vi "grSim_ReplacementTester.vi"(0 "Generate new random points":bool, 1 "IA State":T3, 2 "Atacando contra?":bool, 3 "Test Attacker":bool, 4 "id":i32, 5 "Field defense":i32[](array[numeric]), 6 "Test Mode On":bool, 7 "Number of Points":i32, 9 "Região do campo\nTeste Passe":enum16{"3", "2", "1", "0", "-1", "-2", "-3"}(ring), 10 "Modulo Velocidade":dbl format="%#_13g", 11 "Test Passe":bool, 12 "reset":bool, 13 "Replace Robots":bool) -> (14 "grSim replacement":cluster{"robots":T1[], "ball":T2}, 15 "Replace active":bool, 16 "Number of goals":i16, 18 "kick num":i32, 19 "Completed Generation":bool)   [LabVIEW 2017]
uses:
  Core/AI Input.ctl
  Core/AI Robot.ctl
  Intel/Functions Enum.ctl
  Intel/AttackerStates.ctl
  Path Planning/RRT/PathDests.ctl
  Path Planning/RRT/PathDest.ctl
  Core/AI Ball.ctl
  Core/Field Size.ctl
  Core/AI Judge.ctl
  Intel/Command Enum.ctl
  Util/Events/Events.ctl
  grSim RobotReplacement.ctl
  grSim_BallReplacement.ctl
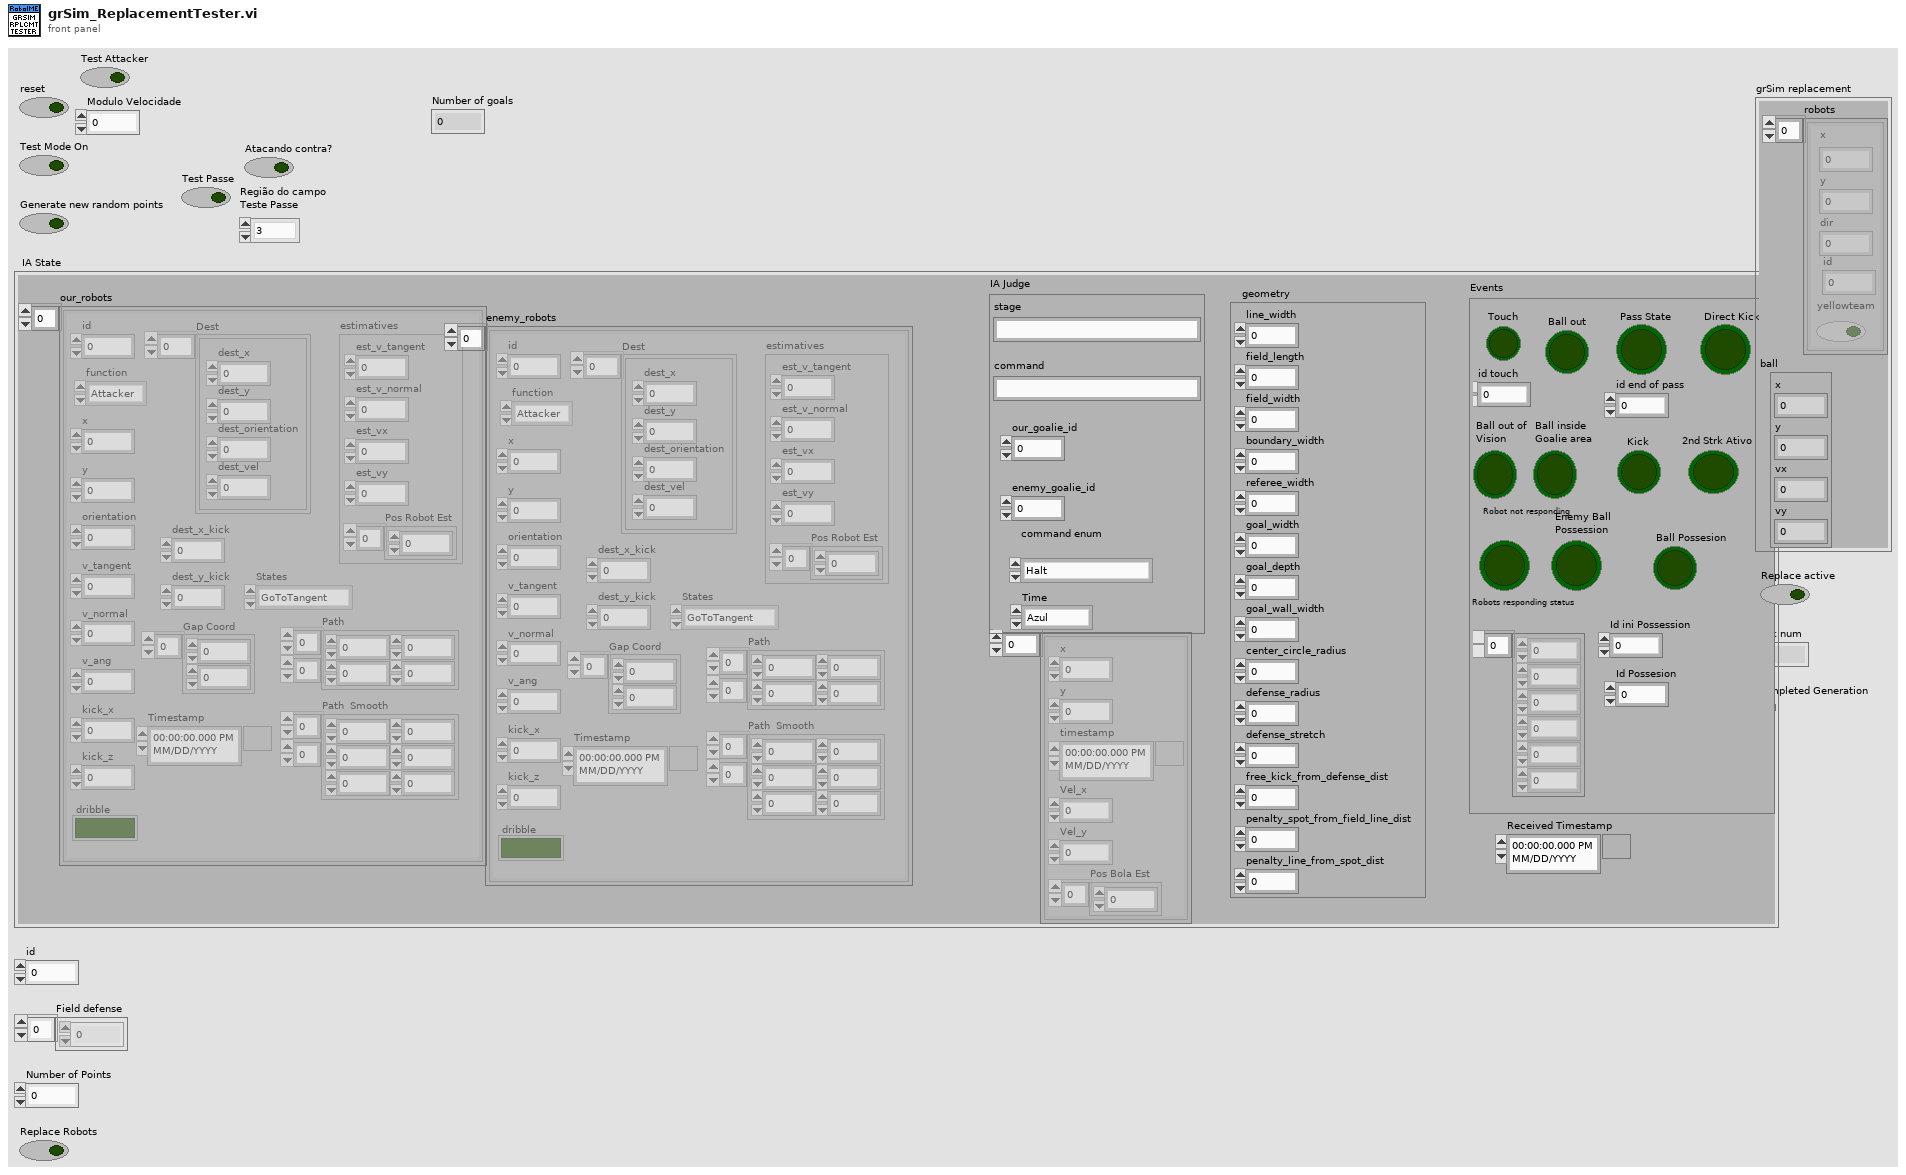
[diagram p1: front panel]
types:
  T1 = typedef "grSim RobotReplacement.ctl" = cluster{"x":dbl, "y":dbl, "dir":dbl, "yellowteam":bool, "id":u32}
  T2 = typedef "grSim_BallReplacement.ctl" = cluster{"x":dbl, "y":dbl, "vx":dbl, "vy":dbl}
  T3 = typedef "AI Input.ctl" = cluster{"our_robots":T4[], "enemy_robots":T4[], "balls":T9[], "geometry":T10, "IA Judge":T11, "Received Timestamp":timestamp, "Events":T13}
  T4 = typedef "AI Robot.ctl" = cluster{"id":u32, "function":T5, "x":dbl, "y":dbl, "orientation":dbl, "v_tangent":dbl, "v_normal":dbl, "v_ang":dbl, "kick_x":dbl, "kick_z":dbl, "dribble":bool, "Timestamp":timestamp, "estimatives":cluster{"est_v_tangent":dbl, "est_v_normal":dbl, "est_vx":dbl, "est_vy":dbl, "Pos Robot Est":dbl[]}, "dest_x_kick":dbl, "dest_y_kick":dbl, "Gap Coord":dbl[], "States":T6, "Path ":dbl[][], "Path  Smooth":dbl[][], "Dest":T7}
  T5 = typedef "Functions Enum.ctl" = enum16{"2nd Striker", "Attacker", "Goalie", "Defender", "Striker", "Goto 0", "Dummy", "Kicker", "ZigZag 0", "ZigZag 1", "ZigZag 2", "ZigZag 3", "ZigZag 4", "ZigZag 5", "ZigZag 6", "ZigZag 7", "ZigZag 8", ""}
  T6 = typedef "AttackerStates.ctl" = enum16{"Pass", "GoToTangent", "BallGetting", "GoToKick", ""}
  T7 = typedef "PathDests.ctl" = T8[]
  T8 = typedef "PathDest.ctl" = cluster{"dest_x":dbl, "dest_y":dbl, "dest_orientation":dbl, "dest_vel":dbl}
  T9 = typedef "AI Ball.ctl" = cluster{"x":dbl, "y":dbl, "timestamp":timestamp, "Vel_x":dbl, "Vel_y":dbl, "Pos Bola Est":dbl[]}
  T10 = typedef "Field Size.ctl" = cluster{"line_width":u32, "field_length":u32, "field_width":u32, "boundary_width":u32, "referee_width":u32, "goal_width":u32, "goal_depth":u32, "goal_wall_width":u32, "center_circle_radius":u32, "defense_radius":u32, "defense_stretch":u32, "free_kick_from_defense_dist":u32, "penalty_spot_from_field_line_dist":u32, "penalty_line_from_spot_dist":u32}
  T11 = typedef "AI Judge.ctl" = cluster{"stage":string, "command":string, "our_goalie_id":dbl, "enemy_goalie_id":dbl, "command enum":T12, "Time":enum16{"Azul", "Amarelo"}}
  T12 = typedef "Command Enum.ctl" = enum16{"Halt", "Stop", "Force Start", "PKA Normal Start", "Prepare Kickoff Ally", "PKE Normal Start", "Prepare Kickoff Enemy", "Prepare Penalty Ally", "PPA Normal Start", "Prepare Penalty Enemy", "PPE Normal Start", "Direct Free Enemy", "Direct Free Ally", "Indirect Free Enemy", "Indirect Free Ally", "Timeout Enemy", "Timeout Ally", "Goal Enemy", "Goal Ally", "Ball Placement Enemy", "Ball Placement Ally", "Normal Half Time", "Extra Time Break", "Extra Half Time", "None", "Post Game"}
  T13 = typedef "Events.ctl" = cluster{"Touch":bool, "Ball out":bool, "id touch":dbl, "Ball out of \nVision":bool, "Ball inside \nGoalie area":bool, "Robot not responding":bool, "Robots responding status":dbl[], "Enemy Ball \nPossession":bool, "Pass State":bool, "id end of pass":dbl, "Kick":bool, "Id ini Possession":dbl, "Ball Possesion":bool, "Id Possesion":dbl, "Direct Kick":bool, "2nd Strk Ativo":bool}
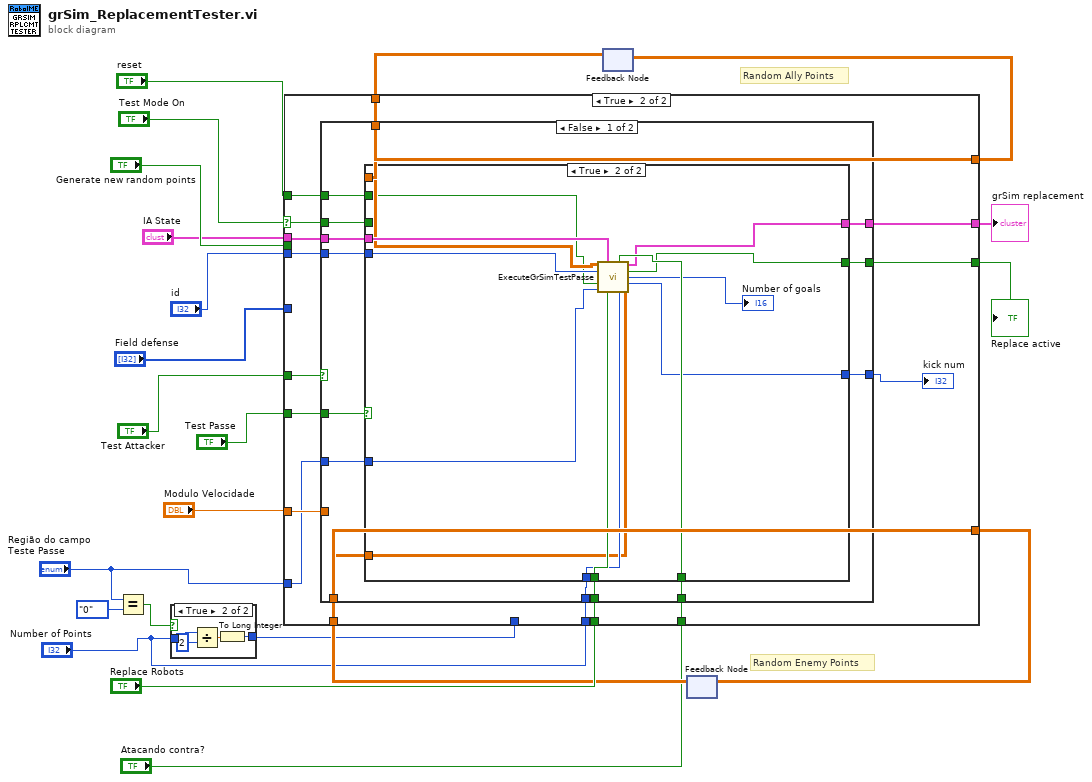
[diagram p0: block diagram]
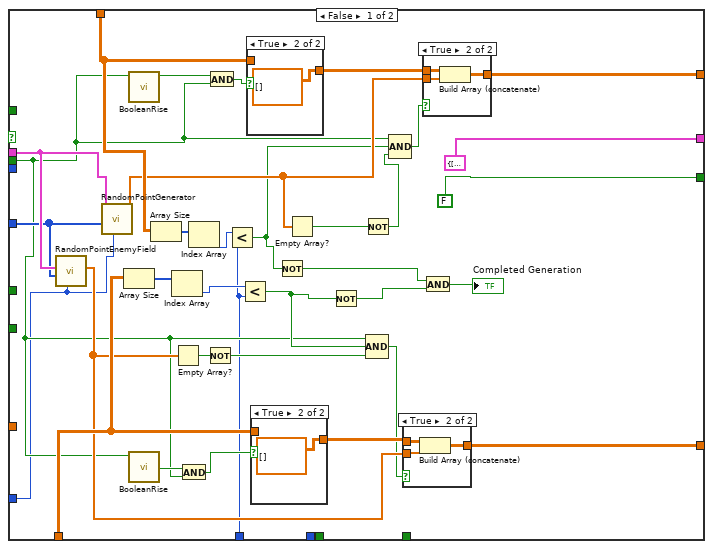
[diagram p3: hidden frame]
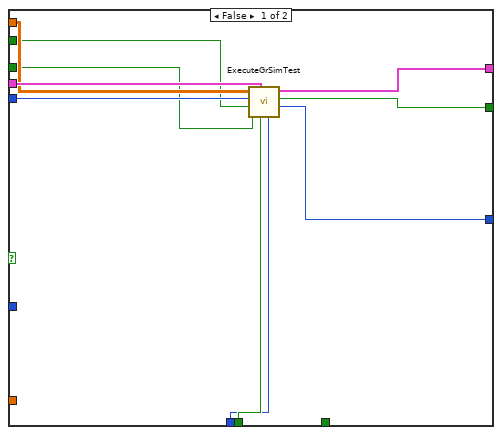
[diagram p8: hidden frame]
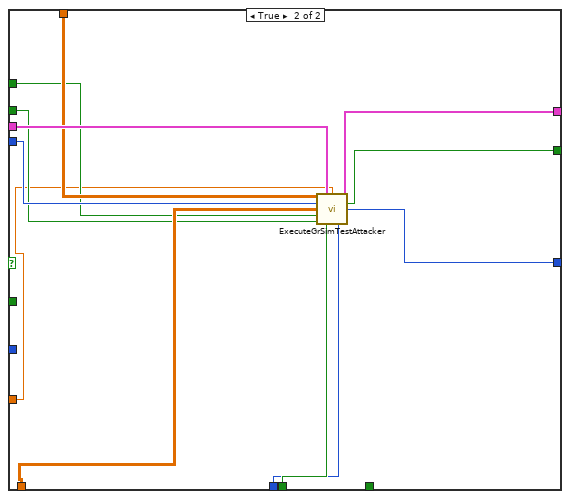
[diagram p9: hidden frame]
diagram:
  # "Random Enemy Points"
  # "Random Ally Points"
  n1 = Equal?(x="Região do campo\nTeste Passe", y=enum16{"3", "2", "1", "0", "-1", "-2", "-3"}."0") -> (x = y?=w3:bool)
  n2 = case shown="True" w3 {
    tunnel: [w23 w24] -> w2
    tunnel: "Number of Points" -> [w23 w27]
    frame False {
    }
    frame True {
      n3 = Divide(x=w27, y=2) -> (x/y=w25:dbl)
      n4 = To Long Integer(number=w25) -> (32bit integer=w24:i32)
    }
  }
  n5 = feedback #1() -> (w19:dbl[][])  [unwired: 1 in]
  n6 = feedback #2() -> (w10:dbl[][])  [unwired: 1 in]
  n7 = case shown="True" "Test Mode On" {
    selector: "Test Mode On" -> [_ w84]
    tunnel: [cluster{"robots":T1[], "ball":T2} {"robots"=[], "ball"={"x"=0.0, "y"=0.0, "vx"=0.0, "vy"=0.0}} ("grSim replacement") w86] -> w12
    tunnel: [FALSE ("Replace active") w87] -> w13
    tunnel: "IA State" -> [w43 w89]
    tunnel: "Field defense" -> [w42 _]
    tunnel: "id" -> [_ w88]
    tunnel: "Generate new random points" -> [w30 _]
    tunnel: [w59 w85] -> w18
    tunnel: w19 -> [w56 w85]
    tunnel: "reset" -> [_ w83]
    tunnel: "Replace Robots" -> [_ w82]
    tunnel: [w44 w79] -> w11
    tunnel: w10 -> [w41 w79]
    tunnel: "Test Attacker" -> [_ w81]
    tunnel: "Modulo Velocidade" -> [_ w80]
    tunnel: "Test Passe" -> [_ w77]
    tunnel: "Atacando contra?" -> [_ w76]
    tunnel: w2 -> [w29 _]
    tunnel: "Região do campo\nTeste Passe" -> [w28 w75]
    tunnel: "Number of Points" -> [_ w74]
    frame False {
      n8 = call "RandomPointEnemyField.vi"("Região do campo\nTeste Passe"=w28, "Field defense"=w42, "IA State Input"=w43) -> ("Point Enemy Field"=w40:dbl[])  [unwired: 8 in]
      n9 = call "RandomPointGenerator.vi"("Região do campo\nTeste Passe"=w28, "Field defense"=w42, "IA State Input"=w43) -> ("Point Ally Field"=w52:dbl[])  [unwired: 8 in]
      n10 = Array Size(array=w41) -> (size(s)=w36:i32[])
      n11 = call "BooleanRise.vi"("Test Mode On"=w30) -> ("Boolean"=w48:bool)  [unwired: 10 in]
      n12 = call "BooleanRise.vi"("Test Mode On"=w30) -> ("Boolean"=w47:bool)  [unwired: 10 in]
      n13 = Array Size(array=w56) -> (size(s)=w54:i32[])
      n14 = Index Array(array=w36) -> (element=w35:i32)  [unwired: 1 in]
      n15 = Empty Array?(array=w40) -> (empty?=w39:bool)
      n16 = And(x=w47, y=w30) -> (x .and. y?=w46:bool)
      n17 = Index Array(array=w54) -> (element=w55:i32)  [unwired: 1 in]
      n18 = Not(x=w39) -> (.not. x?=w38:bool)
      n19 = And(x=w48, y=w30) -> (x .and. y?=w58:bool)
      n20 = Less?(x=w55, y=w29) -> (x < y?=w49:bool)
      n21 = Less?(x=w35, y=w29) -> (x < y?=w34:bool)
      n22 = case shown="True" w58 {
        tunnel: w56 -> [w72 _]
        tunnel: [w72 dbl[][] []] -> w57
        frame False {
        }
        frame True {
        }
      }
      n23 = case shown="True" w46 {
        tunnel: [w66 dbl[][] []] -> w45
        tunnel: w41 -> [w66 _]
        frame False {
        }
        frame True {
        }
      }
      n24 = Not(x=w49) -> (.not. x?=w33:bool)
      n25 = Empty Array?(array=w52) -> (empty?=w50:bool)
      n26 = Not(x=w34) -> (.not. x?=w32:bool)
      n27 = Not(x=w50) -> (.not. x?=w51:bool)
      n28 = Compound Arithmetic op=AND(w30, w34, w38) -> (w37:bool)
      n29 = Compound Arithmetic op=AND(w30, w49, w51) -> (w53:bool)
      n30 = case shown="True" w37 {
        tunnel: [w62 w65] -> w44
        tunnel: w45 -> [w62 w64]
        tunnel: w40 -> [_ w63]
        frame False {
        }
        frame True {
          n31 = Build Array (concatenate)(w64, w63) -> (w65:dbl[][])
        }
      }
      n32 = case shown="True" w53 {
        tunnel: w52 -> [_ w71]
        tunnel: [w68 w70] -> w59
        tunnel: w57 -> [w68 w69]
        frame False {
        }
        frame True {
          n33 = Build Array (concatenate)(w69, w71) -> (w70:dbl[][])
        }
      }
      n34 = And(x=w33, y=w32) -> (x .and. y?=→"Completed Generation":bool)
    }
    frame True {
      n35 = case shown="False" w81 {
        tunnel: w89 -> [w103 w138]
        tunnel: w88 -> [w102 w135]
        tunnel: [w101 w131] -> w87
        tunnel: [w100 w130] -> w86
        tunnel: w85 -> [w99 w137]
        tunnel: w84 -> [w98 w133]
        tunnel: w83 -> [w97 w134]
        tunnel: w82 -> [w96 w132]
        tunnel: w80 -> [_ w128]
        tunnel: w79 -> [w92 w136]
        tunnel: [w95 w129] -> w78
        tunnel: w77 -> [w94 _]
        tunnel: w76 -> [w93 _]
        tunnel: w75 -> [w91 _]
        tunnel: w74 -> [w90 w127]
        frame False {
          n36 = case shown="True" w94 {
            tunnel: w103 -> [w113 w126]
            tunnel: w102 -> [w112 w124]
            tunnel: [w111 w116] -> w101
            tunnel: [w110 w117] -> w100
            tunnel: w99 -> [w109 w125]
            tunnel: w98 -> [w108 _]
            tunnel: w97 -> [w107 w123]
            tunnel: w96 -> [w106 w121]
            tunnel: [w105 w115] -> w95
            tunnel: w93 -> [_ w118]
            tunnel: w92 -> [_ w119]
            tunnel: w91 -> [_ w122]
            tunnel: w90 -> [w104 w120]
            frame False {
              n37 = call "ExecuteGrSimTest.vi"("Number of Points"=w104, "Replace Robots"=w106, "IA State Input"=w113, "Test Mode On"=w108, "reset"=w107, "id"=w112, "RandomAllyPoints"=w109) -> ("kick num"=w105:i32, "Replace active"=w111:bool, "grSim replacement"=w110:cluster{"robots":T1[], "ball":T2})  [unwired: 2 in]
            }
            frame True {
              n38 = call "ExecuteGrSimTestPasse.vi"("RandomAllyPoints"=w125, "IA State Input"=w126, "Atacando contra?"=w118, "id"=w124, "reset"=w123, "Região do campo\nTeste Passe"=w122, "Replace Robots"=w121, "Number of Points"=w120, "RandomEnemyPoints"=w119) -> ("grSim replacement"=w117:cluster{"robots":T1[], "ball":T2}, "Replace active"=w116:bool, "Number of goals"=→"Number of goals":i16, "kick num"=w115:i32)  [unwired: 3 in]
            }
          }
        }
        frame True {
          n39 = call "ExecuteGrSimTestAttacker.vi"("RandomAllyPoints"=w137, "IA State Input"=w138, "Modulo Velocidade"=w128, "id"=w135, "RandomEnemyPoints"=w136, "reset"=w134, "Test Mode On"=w133, "Replace Robots"=w132, "Number of Points"=w127) -> ("grSim replacement"=w130:cluster{"robots":T1[], "ball":T2}, "Replace active"=w131:bool, "kick num"=w129:i32)  [unwired: 4 in]
        }
      }
      "kick num" <- w78
    }
  }
  "Replace active" <- w13
  "grSim replacement" <- w12
  n40 = feedback-in #1(w18) -> ()
  n41 = feedback-in #2(w11) -> ()
